vi "WB10C_conv_W10CB10C_sub.vi"(3 "WB_10C_input":dbl[][](array[numeric])) -> (0 "B_10C":i64[](array[numeric]), 1 "W_10C":i64[][](array[numeric]))   [LabVIEW 2021]
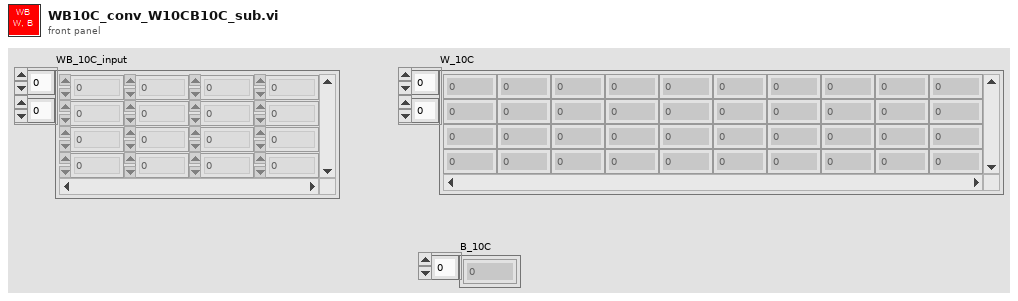
[diagram p1: front panel]
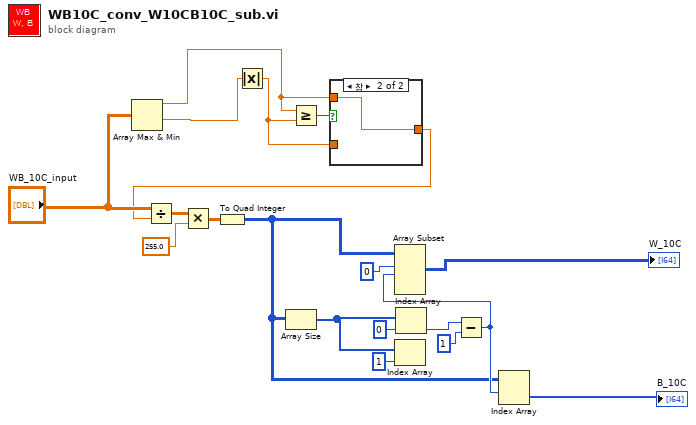
[diagram p0: block diagram]
diagram:
  n1 = Array Max & Min(array="WB_10C_input") -> (max value=w3:dbl, min value=w4:dbl)  [unwired: 2 out]
  n2 = Absolute Value(x=w4) -> (abs(x)=w5:dbl)
  n3 = Greater Or Equal?(x=w3, y=w5) -> (x >= y?=w6:bool)
  n4 = case shown="참" w6 {
    tunnel: [w20 w21] -> w2
    tunnel: w3 -> [_ w21]
    tunnel: w5 -> [w20 _]
    frame False {
    }
    frame True {
    }
  }
  n5 = Divide(x="WB_10C_input", y=w2) -> (x/y=w9:dbl[][])
  n6 = Multiply(x=w9, y=255.0) -> (x*y=w8:dbl[][])
  n7 = To Quad Integer(1:w8) -> (0:w1:i64[][])
  n8 = Array Size(array=w1) -> (size(s)=w17:i32[])
  n9 = Index Array(array=w17, index=1 ("인덱스")) -> ()  [unwired: 1 out]
  n10 = Index Array(array=w17, index=0 ("인덱스")) -> (element=w15:i32)
  n11 = Subtract(x=w15, y=1) -> (x-y=w13:i32)
  n12 = Array Subset(array=w1, index (row)=0 ("인덱스"), length (row)=w13) -> (→"W_10C":i64[][])  [unwired: 2 in]
  n13 = Index Array(array=w1, index (row)=w13) -> (element=→"B_10C":i64[])  [unwired: 1 in]
